vi "Write Time Reference.vi"(8 "error in (no error)":errorcluster, 10 "Report time as result":T1, 11 "Measurement Timer in":refnum<class "Measurement Timer.lvclass">) -> (0 "error out":errorcluster, 3 "Measurement Timer out":refnum<class "Measurement Timer.lvclass">)   [LabVIEW 2015, in "Measurement Timer.lvclass"]
uses:
  Measurement Timer.lvclass
  Log time.ctl
  Measurement Timer.lvclass/Measurement Timer.ctl
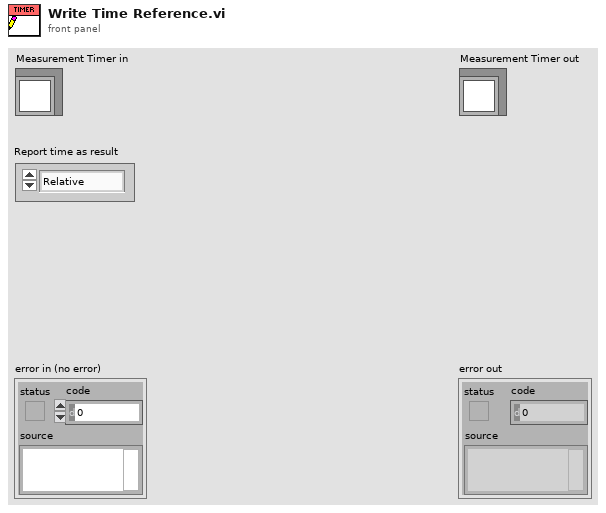
[diagram p1: front panel]
types:
  T1 = typedef "Log time.ctl" = enum16{"Relative", "Absolute", "Do not log"}
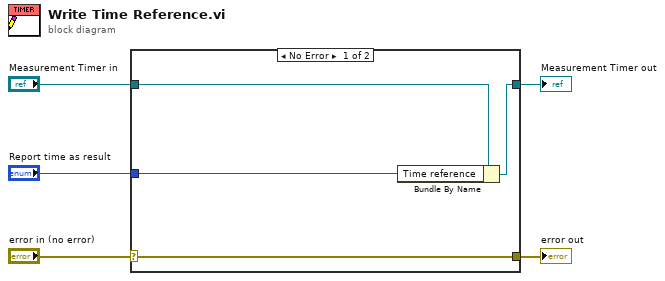
[diagram p0: block diagram]
diagram:
  n1 = case shown="No Error" "error in (no error)" {
    selector: "error in (no error)" -> [w9 w10]
    tunnel: [w9 w10] -> w4
    tunnel: [w7 w11] -> w2
    tunnel: "Measurement Timer in" -> [w8 w11]
    tunnel: "Report time as result" -> [w6 _]
    frame No Error {
      n2 = Bundle By Name(cluster=w8, "Time reference"=w6) -> (w7:refnum<class "Measurement Timer.lvclass">)
    }
    frame Error {
    }
  }
  "error out" <- w4
  "Measurement Timer out" <- w2
